vi "Teardown.vi"(6 "Error":errorcluster, 7 "Actor":refnum<class "Actor.lvclass">, 11 "UnhandledMessages":refnum<class "Msg.lvclass">[](array[class])) -> ()   [LabVIEW 2020, in "_Template.lvlib" / "{{Actor}}.lvlib" / "Actor.lvclass"]
uses:
  Actor.lvclass
  Actor.lvclass/Actor.ctl
  jettl/jettl/Actor/Actor.lvclass
  jettl/jettl/Msg/Msg.lvclass
panel:
  # "This front panel should not be manipulated."
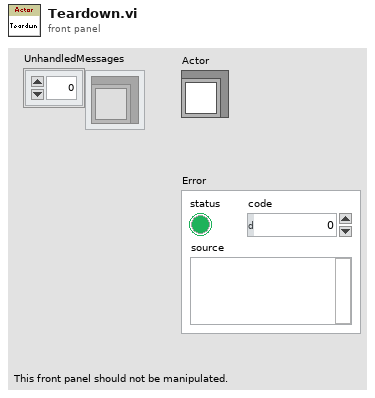
[diagram p1: front panel]
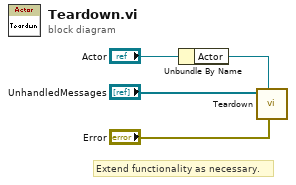
[diagram p0: block diagram]
diagram:
  # "Extend functionality as necessary."
  n1 = Unbundle By Name("Actor") -> ("Actor"=w1:refnum<class "Actor.lvclass">)
  n2 = call-dynamic "Teardown.vi"("Error"="Error", "Actor"=w1, "UnhandledMessages"="UnhandledMessages") -> ()  [unwired: 9 in]
